vi "RM.getResourceTypeArray.vi"() -> (3 "Array":T1[](array[typedef]))   [LabVIEW 2016, in "FPGA Resource Manager.lvlib"]
uses:
  RM.resourceType.ctl
  FPGA Resource Manager.lvlib
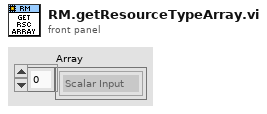
[diagram p1: front panel]
types:
  T1 = typedef "FPGA Resource Manager.lvlib/RM.resourceType.ctl" = enum16{"Scalar Input", "Scalar Output", "Waveform Input", "Waveform Output"}
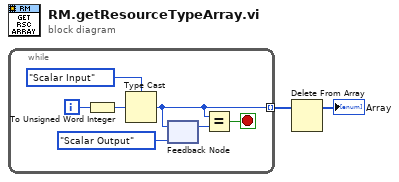
[diagram p0: block diagram]
diagram:
  n1 = while {
    tunnel: [w5] -> w2 mode=indexing
    i -> [w7]
    stop <- w3 stop-if-true
    n2 = To Unsigned Word Integer(number=w7) -> (unsigned 16bit integer=w8:u16)
    n3 = Type Cast(type=RM.resourceType."Scalar Input" ("Resource Type"), x=w8) -> (*(type *) &x=w5:T1)
    n4 = feedback-in #1(w5) -> ()
    n5 = feedback #1(RM.resourceType."Scalar Output" ("Resource Type")) -> (w4:T1)
    n6 = Equal?(x=w5, y=w4) -> (x = y?=w3:bool)
  }
  n7 = Delete From Array(array=w2) -> (array with subset deleted=→"Array":T1[])  [unwired: 2 in, 1 out]
